vi "Configure Offset and Limits (Demodulation - FM).vi"(0 "VISA resource name":refnum<visa-resource-name>, 1 "Carrier Power Upper (10 dBm)":dbl=10.0, 3 "Frequency Dev Upper (100000 Hz)":dbl=100000.0, 5 "Enable Limit (F: Disable)":bool, 9 "Carrier Frequency Offset Upper (1E+6 Hz)":dbl=1000000.0, 11 "error in (no error)":errorcluster, 12 "Frequency Dev Lower (100000 Hz)":dbl=100000.0) -> (4 "VISA resource name out":refnum<visa-resource-name>, 15 "error out":errorcluster)   [LabVIEW 2022 SP3, in "Agilent N934X Series.lvlib"]
doc: "Configures the general setting for FM demodulation offset and limits of Demodulation Option.\n\nNote:\nThis VI is only applicable for N9321C, N9322C, N9323C, N9324C models."
uses:
  <instrlib>/Agilent N934X Series/Agilent N934X Series.lvlib
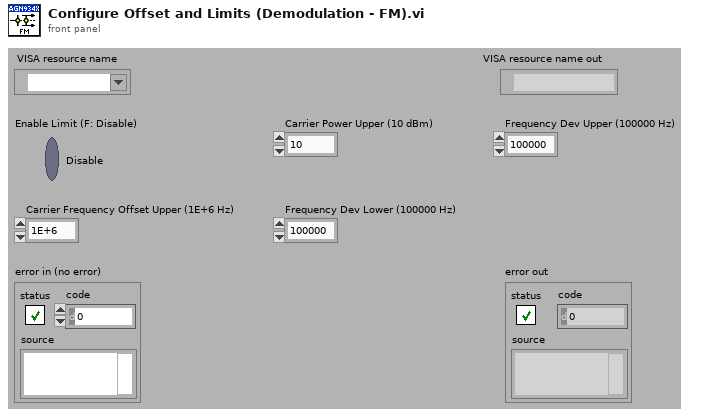
[diagram p1: front panel]
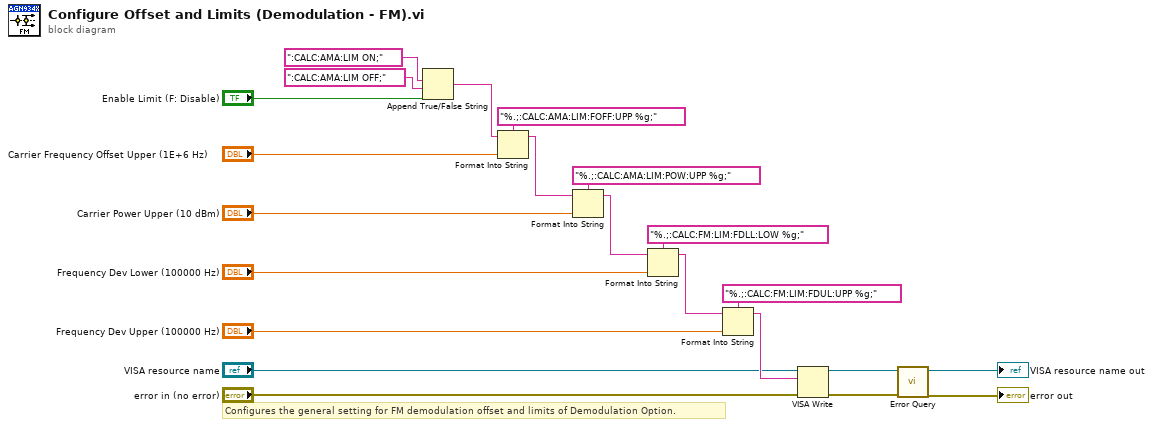
[diagram p0: block diagram]
diagram:
  # "Configures the general setting for FM demodulation offset and limits of Demodulation Option."
  n1 = Append True/False String(1:"Enable Limit (F: Disable)", 2:":CALC:AMA:LIM OFF;", 3:":CALC:AMA:LIM ON;") -> (0:w19:string)  [unwired: 1 in]
  n2 = Format Into String(format string="%.;:CALC:AMA:LIM:FOFF:UPP %g;", initial string=w19, "Carrier Frequency Offset Upper (1E+6 Hz)") -> (resulting string=w16:string)  [unwired: 1 in, 1 out]
  n3 = Format Into String(format string="%.;:CALC:AMA:LIM:POW:UPP %g;", initial string=w16, "Carrier Power Upper (10 dBm)") -> (resulting string=w13:string)  [unwired: 1 in, 1 out]
  n4 = Format Into String(format string="%.;:CALC:FM:LIM:FDLL:LOW %g;", initial string=w13, "Frequency Dev Lower (100000 Hz)") -> (resulting string=w10:string)  [unwired: 1 in, 1 out]
  n5 = Format Into String(format string="%.;:CALC:FM:LIM:FDUL:UPP %g;", initial string=w10, "Frequency Dev Upper (100000 Hz)") -> (resulting string=w7:string)  [unwired: 1 in, 1 out]
  n6 = VISA Write(VISA resource name="VISA resource name", write buffer=w7, error in (no error)="error in (no error)") -> (VISA resource name out=w4:refnum<visa-resource-name>, error out=w3:errorcluster)  [unwired: 1 out]
  n7 = call <instrlib>:"Error Query.vi"("error in (no error)"=w3, "VISA resource name"=w4) -> ("error out"=→"error out":errorcluster, "VISA resource name out"=→"VISA resource name out":refnum<visa-resource-name>)  [unwired: 6 in, 2 out]
